vi "QCA - DUT Close TCP Dll.vi"(0 "CART TCP Connection":refnum<k5>) -> (4 "StatusIsFalse":i16)   [LabVIEW 2012]
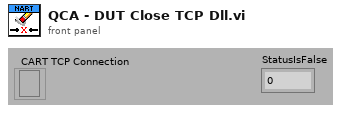
[diagram p1: front panel]
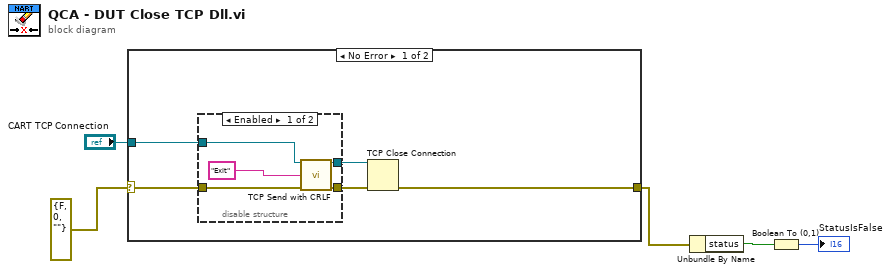
[diagram p0: block diagram]
diagram:
  n1 = case shown="No Error" errorcluster {"status"=FALSE, "code"=0, "source"=""} ("error in (no error)") {
    selector: errorcluster {"status"=FALSE, "code"=0, "source"=""} ("error in (no error)") -> [w10 w18]
    tunnel: [w9 w18] -> w3
    tunnel: "CART TCP Connection" -> [w8 _]
    frame No Error {
      n2 = disable-structure shown="Enabled" {
        disable-tunnel: w10 -> [w15 w16]
        disable-tunnel: w8 -> [w14 w17]
        disable-tunnel: [w13 w16] -> w7
        disable-tunnel: [w12 w17] -> w6
        frame Enabled {
          n3 = call "TCP Send with CRLF.vi"("CART TCP Connection"=w14, "data in"="Exit", "error IO"=w15) -> ("CART TCP Connection Out"=w12:refnum<k5>, "error out"=w13:errorcluster)  [unwired: 11 in]
        }
        frame Disabled {
        }
      }
      n4 = TCP Close Connection(connection ID=w6, error in (no error)=w7) -> (error out=w9:errorcluster)  [unwired: 1 in, 1 out]
    }
    frame Error {
    }
  }
  n5 = Unbundle By Name(w3) -> ("status"=w2:bool)
  n6 = Boolean To (0,1)(Boolean=w2) -> (0, 1=→"StatusIsFalse":i16)
